vi "Intake Controller.vi"(8 "error in":errorcluster) -> ()   [LabVIEW 2018]
doc: "This VI executes continuously carrying out the current operation and responding to updates or new operations. It will often contain the timing or control code that is difficult to place directly in TeleOp. This VI generally opens all sensors and motors and isolates the rest of the robot code from knowing how the operations are carried out."
uses:
  <vilib>/Rock Robotics/WPI/Framework/Completion Status.ctl
  Intake Setpoints.ctl
  Intake Operations.ctl
  <vilib>/Rock Robotics/SystemInterfaces/DIO/FPGA_DIOPWMChannel.ctl
  <vilib>/Rock Robotics/SystemInterfaces/DIO/FPGA_DIOChannel.ctl
  <extravilib>/ChannelInstances/Lossy Stream-bool/Write With Abort.vi
  <extravilib>/ChannelInstances/Lossy Stream-bool/Read With Abort.vi
  <extravilib>/ChannelInstances/Lossy Stream-bool/Endpoint.vi
  <extravilib>/ChannelInstances/Lossy Stream-bool/EndpointRead.vi
  <vilib>/Rock Robotics/WPI/RobotDrive/WPI_RobotDriveOpen2MotorWithSPARK.vi
  <vilib>/Rock Robotics/WPI/Ultrasonic/WPI_SonarMB1010DigitalOpen.vi
  <extravilib>/ChannelInstances/Lossy Stream-bool/Instantiate.vi
  <extravilib>/ChannelInstances/Lossy Stream-bool/)Channel.vi
  <resource>/ChannelSupport/_ChannelSupport/WaitIfNeeded.vi
  Intake Published Globals.vi
  <vilib>/Rock Robotics/WPI/Ultrasonic/WPI_SonarMB1010DigitalGetRange.vi
  <vilib>/Rock Robotics/Network Tables/NT Write Number.vi
  <vilib>/Rock Robotics/Network Tables/NT Write Boolean.vi
  <extravilib>/ChannelInstances/Lossy Stream-bool.lvlib
panel:
  out "Waveform Chart":dbl(graph)=37.89591836734694
  out "Distance":dbl=37.89591836734694
  in  "HasCubeDisance":dbl=9.0
  out "Has Cube":bool
  in  "Interactive Values":T1
  out "Current\nCmd":string="Started at  12:56:38.436\nDefault: Reserve,  S 0.0, D 0.000000"
  in  "Buttons":cluster{"Execute Cmd":bool, "Abort Cmd":bool}
  out "Command Timing":cluster{"Start Time (ms)":u32, "Iterations":i32}={"Start Time (ms)"=8116528, "Iterations"=0}
  out "Status":T3
  # "Tip: It may be helpful to observe inputs and sensor values.\nYou may also want to display tuning or debugging controls."
  # "Interactive Command: You may fill in the settings for a command\nand schedule it with the Execute button. You can observe and abort\nany command while fine tuning the code for the controller."
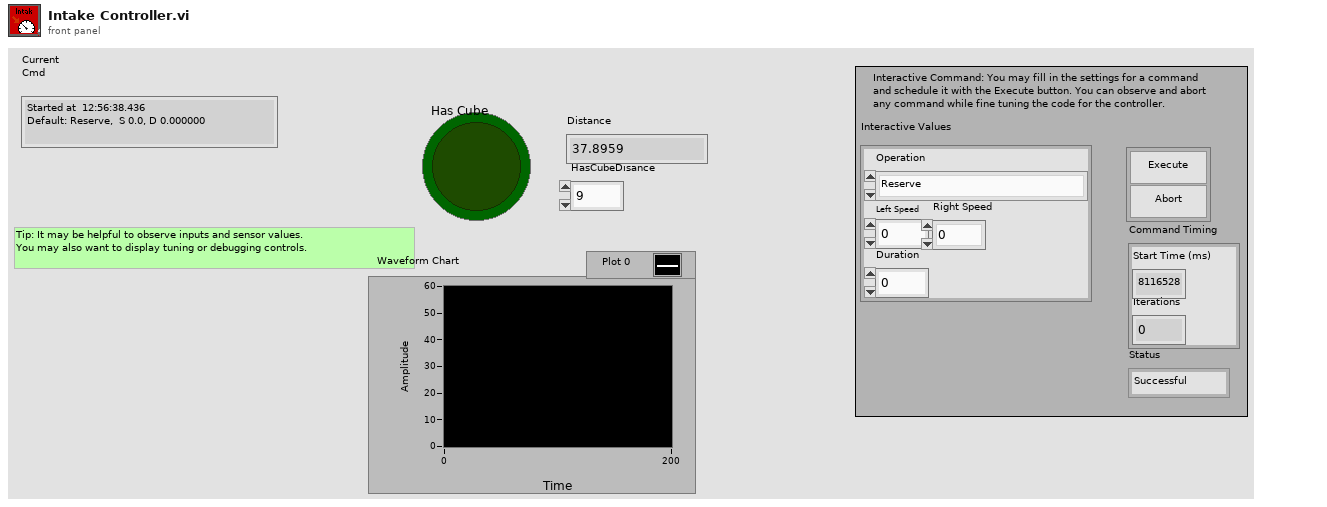
[diagram p1: front panel]
types:
  T1 = typedef "Intake Setpoints.ctl" = cluster{"Operation":T2, "Left Speed":dbl, "Duration":dbl, "Right Speed":dbl}
  T2 = typedef "Intake Operations.ctl" = enum16{"Reserve", "Read Current", "Immediate", "Intake for Duration", "Intake Until Cube"}
  T3 = typedef "Completion Status.ctl" = enum16{"Successful", "Aborted", "Incomplete"}
  T4 = typedef "FPGA_DIOChannel.ctl" = enum8{"DIO 0", "DIO 1", "DIO 2", "DIO 3", "DIO 4", "DIO 5", "DIO 6", "DIO 7", "DIO 8", "DIO 9", "DIO MXP 0", "DIO MXP 1", "DIO MXP 2", "DIO MXP 3", "DIO MXP 4", "DIO MXP 5", "DIO MXP 6", "DIO MXP 7", "DIO MXP 8", "DIO MXP 9", "DIO MXP 10", "DIO MXP 11", "DIO MXP 12", "DIO MXP 13", "DIO MXP 14", "DIO MXP 15", "SPI Port CS1", "SPI Port CS2", "SPI Port CS3", "SPI Port MISO", "SPI Port MOSI", "Invalid"}
  T5 = typedef "FPGA_DIOPWMChannel.ctl" = enum8{"PWM 0", "PWM 1", "PWM 2", "PWM 3", "PWM 4", "PWM 5", "PWM 6", "PWM 7", "PWM 8", "PWM 9", "PWM MXP 0", "PWM MXP 1", "PWM MXP 2", "PWM MXP 3", "PWM MXP 4", "PWM MXP 5", "PWM MXP 6", "PWM MXP 7", "PWM MXP 8", "PWM MXP 9", "Invalid"}
  T6 = typedef "WPI_SonarMB1010DigitalDeviceRef.ctl" = cluster{"CounterDevRef":T7, "Scaling factor (s/in)":dbl}
  T7 = typedef "WPI_CounterDevRef.ctl" = cluster{"DevStatus":errorcluster, "CntIndex":T8}
  T8 = typedef "FPGA_CounterCtrSystemIndex.ctl" = enum8{"Ctr 0", "Ctr 1", "Ctr 2", "Ctr 3", "Ctr 4", "Ctr 5", "Ctr 6", "Ctr 7", "Invalid"}
  T9 = typedef "WPI_RobotDriveDevRef.ctl" = cluster{"DevStatus":errorcluster, "Motors[]":T10[], "Square Inputs":bool, "Max Output":dbl}
  T10 = typedef "WPI_MotorControlDeviceRef.ctl" = cluster{"DeviceStatus":errorcluster, "Type":T11, "PWM":cluster{"PWM Channel":T5, "DeadBand":T12}, "CAN":cluster{"Device Number":u8, "SetOutput VI Ref":variant, "GetOutput VI Ref":variant, "Enable VI Ref":variant, "Disable VI Ref":variant, "Data":variant}, "Invert":bool, "DIO PWM":cluster{"PWM \"Enable\" Channel":T5, "DIOChannel":T4, "PWM Rate":dbl}}
  T11 = typedef "WPI_MotorControlType.ctl" = enum16{"PWM", "CAN", "DIO PWM"}
  T12 = typedef "WPI_PWMDeadband.ctl" = cluster{"Name":string, "maxPositivePwm":i32, "minPositivePwm":i32, "centerPwm":i32, "maxNegativePwm":i32, "minNegativePwm":i32, "angularRange":u16}
  T13 = typedef "Lossy Stream-bool.lvlib/)Channel.ctl" = refnum<queue>
  T14 = typedef "Command Status Info.ctl" = cluster{"Name":string, "Status":T3, "notifier out":T15}
  T15 = typedef "Completion Notifier.ctl" = refnum<notifier>
  T16 = cluster{"Current Command":T1, "Command Timing":cluster{"Start Time (ms)":u32, "Iterations":i32}, "Command Arguments":cluster{"Command Info":T14, "Description":string, "Default Command":T1, "queue out":refnum<queue>, "Subsystem Name":string}}
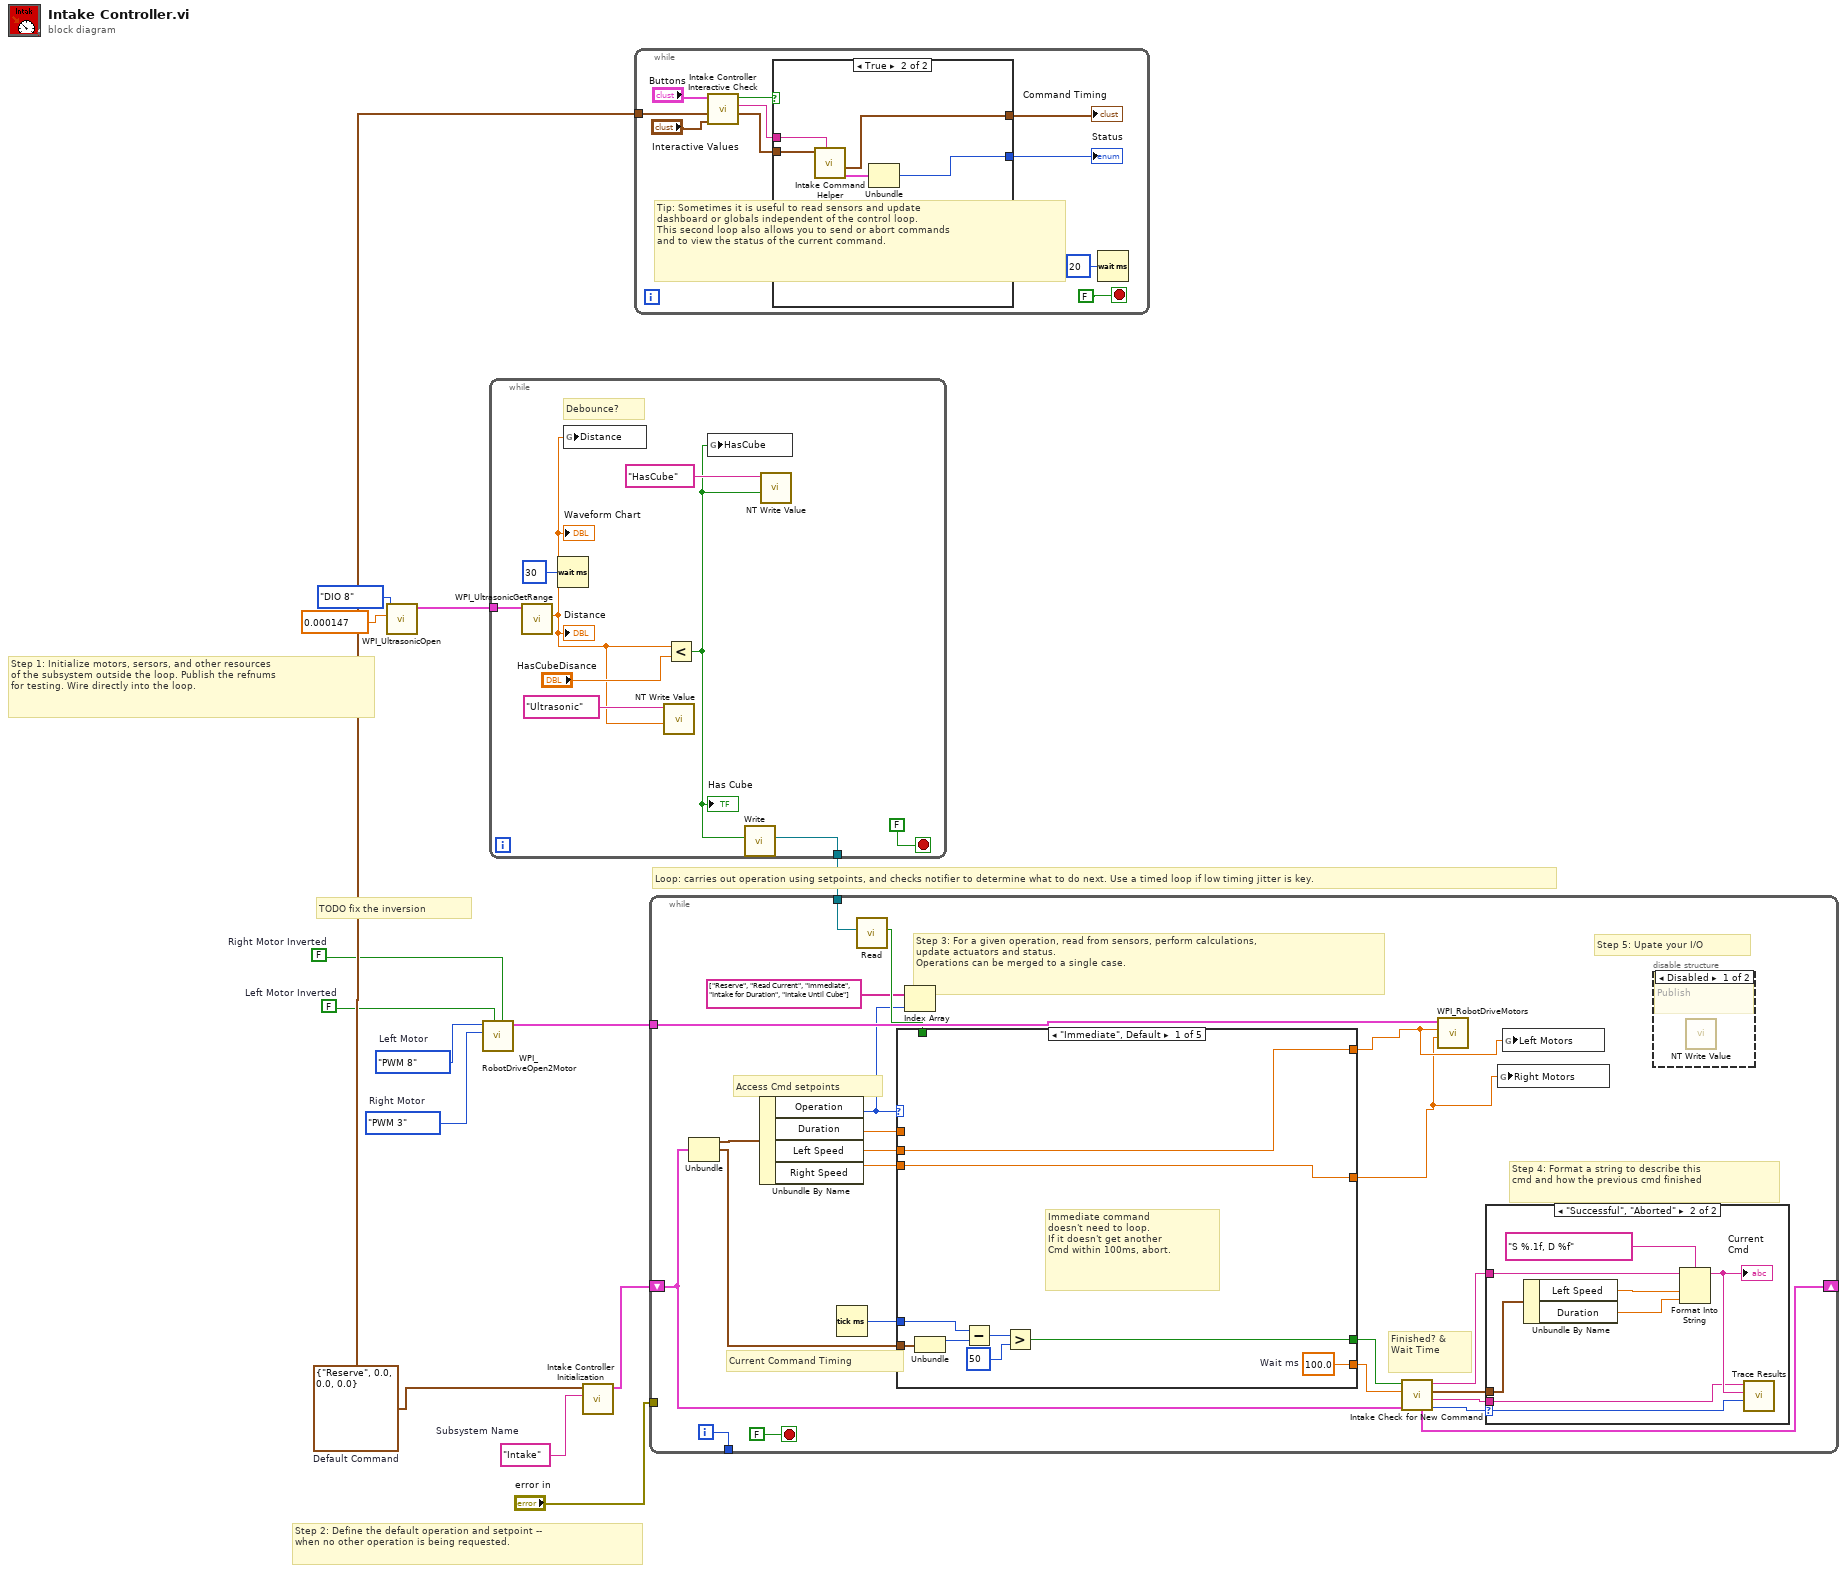
[diagram p0: block diagram]
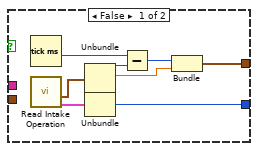
[diagram p2: hidden frame]
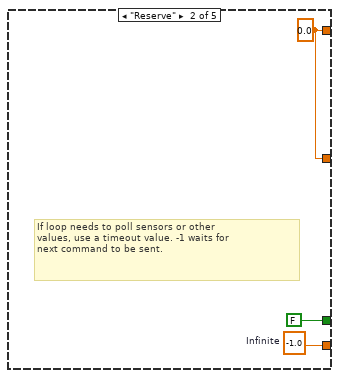
[diagram p3: hidden frame]
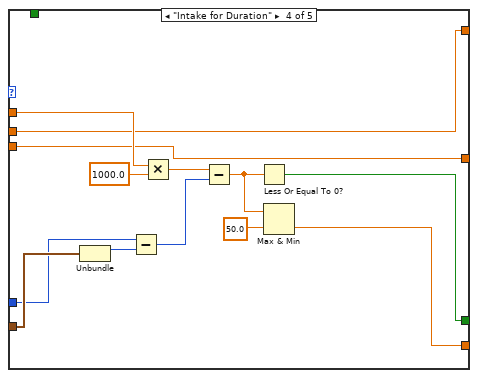
[diagram p5: hidden frame]
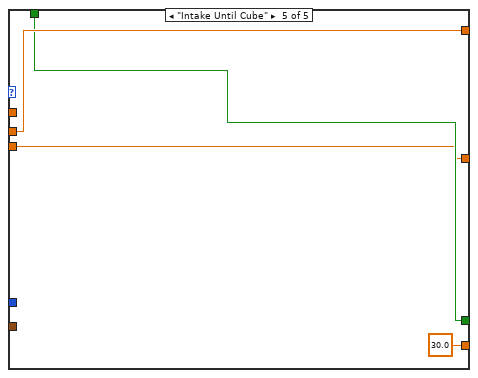
[diagram p6: hidden frame]
diagram:
  w4 = FALSE  # Left Motor Inverted
  w7 = FALSE  # Right Motor Inverted
  w5 = FPGA_DIOPWMChannel."PWM 3"  # Right Motor
  w6 = FPGA_DIOPWMChannel."PWM 8"  # Left Motor
  w10 = T1 {"Operation"=enum."Reserve", "Left Speed"=0.0, "Duration"=0.0, "Right Speed"=0.0}  # Default Command
  w11 = "Intake"  # Subsystem Name
  # "Step 2: Define the default operation and setpoint --\nwhen no other operation is being requested."
  # "TODO fix the inversion"
  # "Tip: Sometimes it is useful to read sensors and update\ndashboard or globals independent of the control loop.\nThis second loop also allows you to send or abort commands\nand to view the status of the current command."
  # "Step 1: Initialize motors, sersors, and other resources\nof the subsystem outside the loop. Publish the refnums\nfor testing. Wire directly into the loop."
  # "Loop: carries out operation using setpoints, and checks notifier to determine what to do next. Use a timed loop if low timing jitter is key."
  n1 = call-poly <vilib>:"WPI_UltrasonicOpen.vi"("Scaling factor (s/in)"=0.000147, "DIO Channel"=FPGA_DIOChannel."DIO 8") -> ("SonarMB1010DigitalDevRef"=w3:T6)  [unwired: 8 in, 1 out]
  n2 = call-poly <vilib>:"WPI_RobotDriveOpen2Motor.vi"("Right Motor Inverted"=w7, "Left Motor Inverted"=w4, "Right Motor"=w5, "Left Motor"=w6) -> ("RobotDriveDevRef"=w8:T9)  [unwired: 6 in, 1 out]
  n3 = while {
    tunnel: w3 -> [w18]
    tunnel: [w21] -> w9
    stop <- FALSE stop-if-true
    # "Debounce?"
    n4 = call-poly <vilib>:"WPI_UltrasonicGetRange.vi"("SonarMB1010DigitalDevRef"=w18) -> ("Distance"=w14:dbl)  [unwired: 8 in, 2 out]
    "Distance" <- w14
    "Waveform Chart" <- w14
    n5 = Wait (ms)(milliseconds to wait=u32 30) -> ()  [unwired: 1 out]
    n6 = global write "Intake Published Globals.vi" "Distance"(w14) -> ()
    n7 = call-poly <vilib>:"NT Write Value.vi"("Numeric"=w14, "Name"="Ultrasonic") -> ()  [unwired: 9 in, 1 out]
    n8 = Less?(x=w14, y="HasCubeDisance") -> (x < y?=w16:bool)
    "Has Cube" <- w16
    n9 = global write "Intake Published Globals.vi" "HasCube"(w16) -> ()
    n10 = call <extravilib>:"Write.vi"("element"=w16) -> ("channel"=w21:T13)  [unwired: 8 in, 2 out]
    n11 = call-poly <vilib>:"NT Write Value.vi"("Boolean"=w16, "Name"="HasCube") -> ()  [unwired: 9 in, 1 out]
  }
  n12 = call "Intake Controller Initialization.vi"("Subsystem Name"=w11, "Default Command"=w10) -> ("Current Command"=w12:T16)  [unwired: 9 in]
  n13 = while {
    tunnel: w10 -> [w29]
    stop <- FALSE stop-if-true
    n14 = call "Intake Controller Interactive Check.vi"("Interactive Command in"="Interactive Values", "Default Command"=w29, "Buttons"="Buttons") -> ("Interactive Command out"=w26:T1, "Trace String"=w27:string, "Schedule"=w28:bool)  [unwired: 6 in]
    n15 = case shown="True" w28 {
      tunnel: [w40 w45] -> w25
      tunnel: w26 -> [_ w43]
      tunnel: [w36 w41] -> w24
      tunnel: w27 -> [_ w44]
      frame False {
        n16 = Tick Count (ms)() -> (millisecond timer value=w35:u32)
        n17 = call "Read Intake Operation.vi"() -> ("Command Info"=w33:T14, "SubSystem Data"=w34:T1)  [unwired: 9 in, 1 out]
        n18 = Unbundle(w34) -> ("Operation"=w39:T2, "Left Speed"=w37:dbl)  [unwired: 2 out]
        n19 = Unbundle(w33) -> ("Status"=w40:T3)  [unwired: 2 out]
        n20 = Subtract(x=w35, y=w39) -> (x-y=w38:u32)
        n21 = Bundle(w38, "Left Speed"=w37) -> (w36:cluster{u32, "Left Speed":dbl})  [unwired: 1 in]
      }
      frame True {
        n22 = call "Intake Command Helper.vi"("Description"=w44, "SubSystem Data"=w43) -> ("Command Info Out"=w42:T14, "Command Timing"=w41:cluster{"Start Time (ms)":u32, "Iterations":i32})  [unwired: 7 in, 1 out]
        n23 = Unbundle(w42) -> ("Status"=w45:T3)  [unwired: 2 out]
      }
    }
    "Status" <- w25
    "Command Timing" <- w24
    n24 = Wait (ms)(milliseconds to wait=u32 20) -> ()  [unwired: 1 out]
  }
  n25 = while {
    shift-right: [w61] -> _
    shift-left: w12 -> [w54]
    tunnel: [w67] -> _
    tunnel: "error in" -> [_]
    tunnel: w8 -> [w53]
    tunnel: w9 -> [w52]
    i -> [w67]
    stop <- FALSE stop-if-true
    # "Step 5: Upate your I/O"
    # "Step 4: Format a string to describe this\ncmd and how the previous cmd finished"
    # "Current Command Timing"
    # "Access Cmd setpoints"
    # "Finished? &\nWait Time"
    # "Step 3: For a given operation, read from sensors, perform calculations,\nupdate actuators and status.\nOperations can be merged to a single case."
    n26 = Unbundle(w54) -> ("Current Command"=w66:T1, "Command Timing"=w63:cluster{"Start Time (ms)":u32, "Iterations":i32})  [unwired: 1 out]
    n27 = Unbundle By Name(w66) -> ("Operation"=w50:T2, "Duration"=w65:dbl, "Left Speed"=w62:dbl, "Right Speed"=w48:dbl)
    n28 = Tick Count (ms)() -> (millisecond timer value=w64:u32)
    n29 = call <extravilib>:"Read.vi"("channel"=w52) -> ("element"=w51:bool)  [unwired: 5 in, 5 out]
    n30 = case shown="\"Immediate\", Default" w50 {
      tunnel: [w77 w80 _ w84 30.0 ("Infinite")] -> w59
      tunnel: [w71 FALSE ("ignore previous (F)") _ w85 w95] -> w60
      tunnel: w63 -> [w73 _ _ w83 _]
      tunnel: w65 -> [_ _ _ w87 _]
      tunnel: w64 -> [w72 _ _ w82 _]
      tunnel: w62 -> [w70 _ _ w86 w97]
      tunnel: [w70 w78 _ w86 w97] -> w47
      tunnel: w51 -> [_ _ _ _ w95]
      tunnel: [w69 w78 _ w81 w94] -> w46
      tunnel: w48 -> [w69 _ _ w81 w94]
      frame "Immediate", Default {
        w77 = 100.0  # Wait ms
        # "Immediate command\ndoesn't need to loop.\nIf it doesn't get another\nCmd within 100ms, abort."
        n31 = Unbundle(w73) -> ("Start Time (ms)"=w76:u32)  [unwired: 1 out]
        n32 = Subtract(x=w72, y=w76) -> (x-y=w75:u32)
        n33 = Greater?(x=w75, y=u8 50 ("Left Motor")) -> (0:w71:bool)
      }
      frame "Reserve" {
        w78 = 0.0 ("Speed")
        w80 = -1.0  # Infinite
        # "If loop needs to poll sensors or other\nvalues, use a timeout value. -1 waits for\nnext command to be sent."
      }
      frame "Read Current" {
      }
      frame "Intake for Duration" {
        n34 = Unbundle(w83) -> ("Start Time (ms)"=w90:u32)  [unwired: 1 out]
        n35 = Subtract(x=w82, y=w90) -> (x-y=w93:u32)
        n36 = Multiply(x=w87, y=1000.0) -> (x*y=w92:dbl)
        n37 = Subtract(x=w92, y=w93) -> (x-y=w89:dbl)
        n38 = Less Or Equal To 0?(x=w89) -> (x <= 0?=w85:bool)
        n39 = Max & Min(x=w89, y=50.0) -> (min(x,y)=w84:dbl)  [unwired: 1 out]
      }
      frame "Intake Until Cube" {
      }
    }
    n40 = Index Array(array=string[] ["Reserve", "Read Current", "Immediate", "Intake for Duration", "Intake Until Cube"] ("Strings []"), index=w50) -> ()  [unwired: 1 out]
    n41 = call "Intake Check for New Command.vi"("Current Command"=w54, "Wait time (ms)"=w59, "Finished?"=w60) -> ("Completion"=w55:T3, "Subsystem Name"=w56:string, "Current Command"=w57:T1, "Initial Trace String"=w58:string, "NextCommand"=w61:T16)  [unwired: 4 in]
    n42 = call <vilib>:"WPI_RobotDriveMotors.vi"("RightSpeed"=w46, "LeftSpeed"=w47, "RobotDriveDevRef"=w53) -> ()  [unwired: 1 in, 8 out]
    n43 = case shown="\"Successful\", \"Aborted\"" w55 {
      selector: w55 -> [_ w105]
      tunnel: w58 -> [_ w101]
      tunnel: w57 -> [_ w102]
      tunnel: w56 -> [_ w98]
      frame "Incomplete", Default {
        # "Continuing current command"
      }
      frame "Successful", "Aborted" {
        # "Report and setup for next command"
        n44 = Unbundle By Name(w102) -> ("Left Speed"=w104:dbl, "Duration"=w99:dbl)
        n45 = Format Into String(format string="S %.1f, D %f", initial string=w101, w104, w99) -> (resulting string=w100:string)  [unwired: 1 in, 1 out]
        "Current\nCmd" <- w100
        n46 = call <vilib>:"Trace Results.vi"("Status of previous command"=w105, "Description"=w100, "Subsystem"=w98) -> ()  [unwired: 9 in]
      }
    }
    n47 = global write "Intake Published Globals.vi" "Right Motors"(w46) -> ()
    n48 = global write "Intake Published Globals.vi" "Left Motors"(w47) -> ()
    n49 = disable-structure shown="Disabled" {
      frame Disabled {
        # "Publish"
        n50 = call-poly <vilib>:"NT Write Value.vi"() -> ()  [unwired: 11 in, 1 out]
      }
      frame Enabled {
      }
    }
  }
